vi "5492_GetTargetAngle.vi"() -> (3 "Target Angle":dbl)   [LabVIEW 2016]
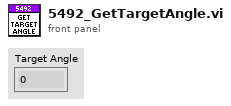
[diagram p1: front panel]
types:
  T1 = cluster{"centerX":dbl[], "centerY":dbl[], "area":dbl[], "width":dbl[], "height":dbl[], "solidity":dbl[]}
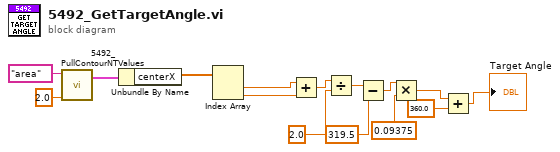
[diagram p0: block diagram]
diagram:
  n1 = call "5492_PullContourNTValues.vi"("Shapes Found"=2.0, "Max Value\nMax Value"="area" ("Max Value\nMax Value")) -> ("Output Cluster"=w13:T1)  [unwired: 9 in]
  n2 = Unbundle By Name(w13) -> ("centerX"=w12:dbl[])
  n3 = Index Array(array=w12) -> (element #1=w11:dbl, element #2=w10:dbl)  [unwired: 2 in]
  n4 = Add(x=w11, y=w10) -> (x+y=w9:dbl)
  n5 = Divide(x=w9, y=2.0) -> (x/y=w6:dbl)
  n6 = Subtract(x=w6, y=319.5) -> (x-y=w4:dbl)
  n7 = Multiply(x=w4, y=0.09375) -> (x*y=w2:dbl)
  n8 = Add(x=w2, y=360.0) -> (x+y=→"Target Angle":dbl)
